vi "Get Display Name.vi"(8 "error in (no error)":errorcluster, 11 "Error in":refnum<class "Error.lvclass">) -> (0 "error out":errorcluster, 2 "localized name":string, 3 "Error out":refnum<class "Error.lvclass">)   [LabVIEW 2009, in "NavScreen.lvlib" / "Error.lvclass"]
uses:
  Error.lvclass
  ClickableText/ClickableText.lvclass
panel:
  in  "format string":string="ERROR - %s"
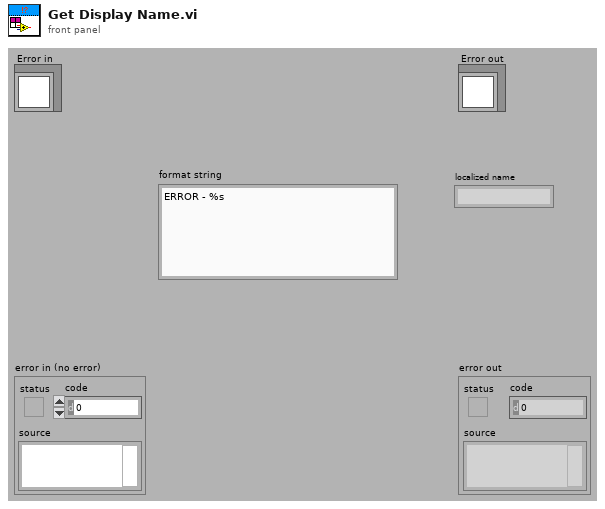
[diagram p1: front panel]
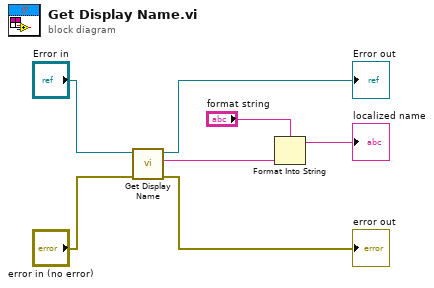
[diagram p0: block diagram]
diagram:
  n1 = call-parent "Get Display Name.vi"("error in (no error)"="error in (no error)", "ClickableText in"="Error in") -> ("error out"=→"error out":errorcluster, "localized name"=w2:string, "ClickableText out"=→"Error out":refnum<class "Error.lvclass">)  [unwired: 7 in]
  n2 = Format Into String(format string="format string", w2) -> (resulting string=→"localized name":string)  [unwired: 2 in, 1 out]
